vi "1_SimpleDemo_TH260Histo.vi"() -> ()   [LabVIEW 2017]
uses:
  _lib/PQ/TimeHarp260/TH260_MeasMode.ctl
  _lib/PQ/TimeHarp260/TH260_TimingMode.ctl
  _lib/PQ/TimeHarp260/th260lib_x86_x64_UIThread.llb/TH260_DllPath_global.vi
  <vilib>/Utility/error.llb/Error Cluster From Error Code.vi
  _lib/PQ/TimeHarp260/TH260_LibVersion_global.vi
  <vilib>/ErrorRing/Error Ring.xnode
panel:
  in  "dtcode":i32(ring) caption="Deadtime  [ns]" items=["24", "44", "66", "88", "112", "135", "160", "180"]
  in  "TrgLevel":i32=-100 caption="Trg.Level [mV]" min=-1200 max=1200 step=1
  in  "TrgEdge":i32(ring) items=["falling", "rising"]
  in  "SyncTrgEdge":i32(ring) caption="TrgEdge" items=["falling", "rising"]
  in  "SyncTrgLevel":i32=-100 caption="Trg.Level [mV]" min=-1200 max=1200 step=1
  in  "Binning":i32(ring) caption="Resolution [ps]" items=["25.000000", "50.000000", "100.000000", "200.000000", "400.000000", "800.000000", "1600.000000", "3200.000000", "6400.000000", "12800.000000", "25600.000000", "51200.000000", "102400.000000", "204800.000000", "409600.000000", "819200.000000", "1638400.000000", "3276800.000000", "6553600.000000", "13107200.000000", "26214400.000000", "52428800.000000"]
  in  "HistoLength":i32(ring)=5 caption="Histo Length" items=["1024", "2048", "4096", "8192", "16384", "32768"]
  in  "Acqu.Time":i32=10000 caption="Acqu.Time [ms]" min=1 max=360000000 step=1
  in  "GlobalOffset":i32 caption="GlobalOffset [ns]" min=0 max=100000000 step=1
  in  "OverflowLevel":u32=65535 min=1 step=1
  in  "StopOnOverflow":bool=TRUE
  in  "InputZeroX":i32=-10 caption="ZeroCr. [mV]" min=-40 max=0 step=1
  in  "InputCFDLevel":i32=-100 caption="CFDLevel [mV]" min=-1200 max=0 step=1
  in  "Offset":i32 caption="Offset [ps]" min=-99999 max=99999 step=1
  in  "Enable":bool=TRUE
  in  "SyncZeroX":i32=-10 caption="ZeroCr. [mV]" min=-40 max=0 step=1
  in  "SyncCFDLevel":i32=-100 caption="CFDLevel [mV]" min=-1200 max=0 step=1
  in  "SyncOffset":i32 caption="SyncOffset [ps]" min=-99999 max=99999 step=1
  in  "SyncDivider":i32(ring)=8 items=["1"=1, "2"=2, "4"=4, "8"=8]
  out "HistoGraph":T1(graph)={0.0, "Resolution"=0.025, "Histogram"=array2x32768[65536 elements]}
  out "CountRates":i32[](array[numeric]) caption="Count Rates [cps]"
  out "SyncRate":i32 caption="Sync Rate [cps]"
  in  "stop":bool
  out "error out":errorcluster
  # "Acquisition"
  # "All Channels"
  # "Sync"
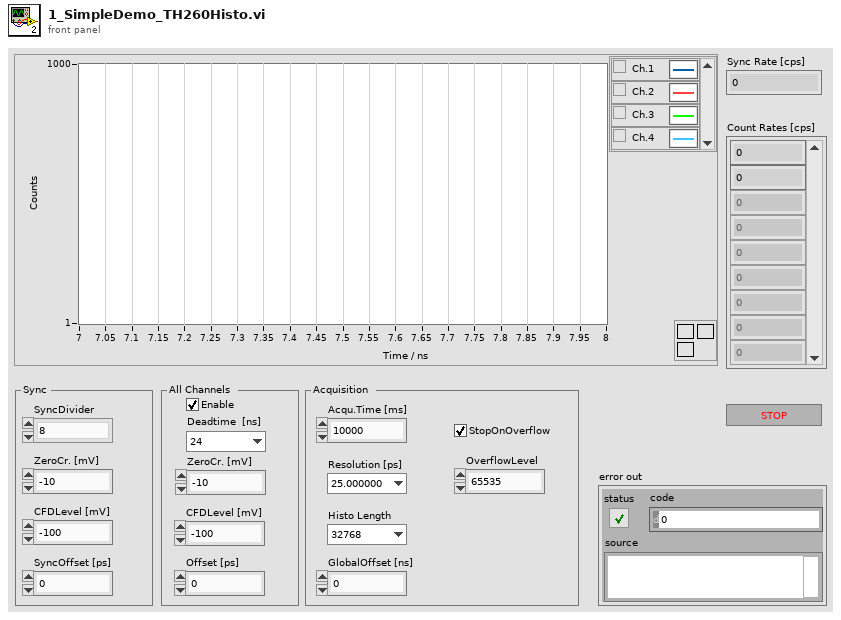
[diagram p1: front panel]
types:
  T1 = cluster{dbl, "Resolution":dbl, "Histogram":u32[][]}
  T2 = typedef "TH260_TimingMode.ctl" = i32
  T3 = typedef "TH260_MeasMode.ctl" = i32
  T4 = typedef "TH260_InitInfo.ctl" = cluster{"Library Version":string, "Serial No.":string, "Model":string, "Partnum":string, "Version":string, "features":i32, "nchannels":i32, "Base Resolution":dbl, "Bin Steps":i32}
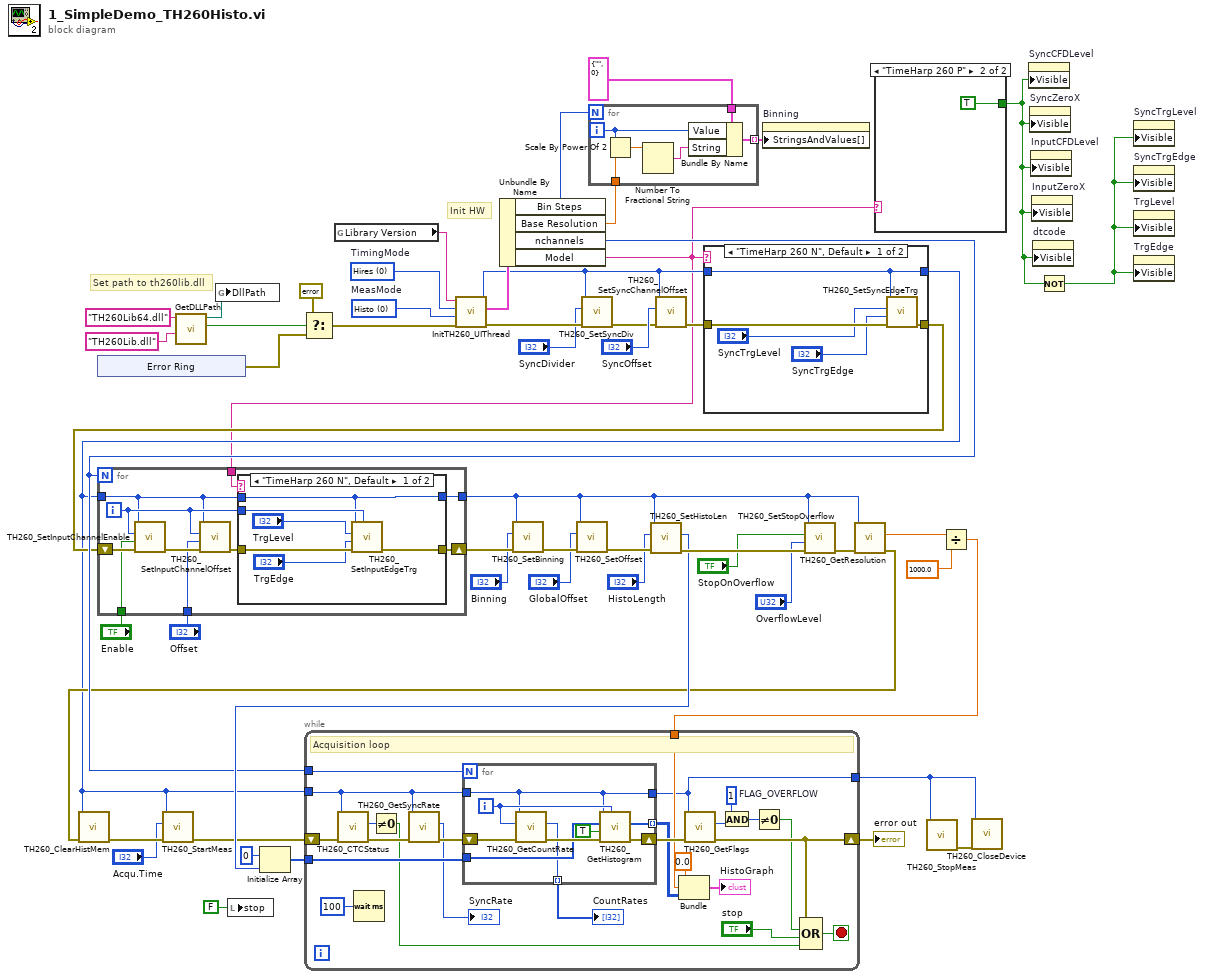
[diagram p0: block diagram]
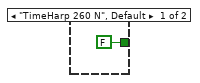
[diagram p2: hidden frame]
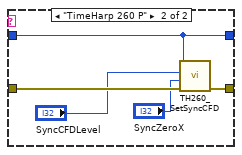
[diagram p3: hidden frame]
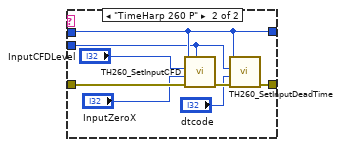
[diagram p4: hidden frame]
diagram:
  w4 = T2 0 items=["Hires", "Lowres"]  # TimingMode
  w54 = T3 0 items=["Histo"=0, "T2"=2, "T3"=3]  # MeasMode
  # "Init HW"
  # "Set path to th260lib.dll"
  n1 = xnode "Error Ring"() -> ("error out"=w53:errorcluster)
  n2 = call "GetDLLPath.vi"("DllName_32bit"="TH260Lib.dll" ("name or relative path"), "DllName_64bit"="TH260Lib64.dll" ("name or relative path")) -> ("file exists?"=w51:bool, "DLLPath"=w50:path)  [unwired: 8 in]
  n3 = global write "TH260_DllPath_global.vi" "DllPath"(w50) -> ()
  n4 = local write "stop"(FALSE ("stop")) -> ()
  n5 = Select(t=errorcluster {"status"=FALSE, "code"=0, "source"=""} ("error IO"), s=w51, f=w53) -> (s? t:f=w47:errorcluster)
  n6 = global read "TH260_LibVersion_global.vi" "Library Version"() -> (w12:string)
  n7 = call "InitTH260_UIThread.vi"("error in (no error)"=w47, "MeasMode"=w54, "TimingMode"=w4, "Library Version"=w12) -> ("error out"=w42:errorcluster, "Init Info"=w44:T4, "DevIdx"=w16:i32)  [unwired: 5 in]
  n8 = Unbundle By Name(w44) -> ("Bin Steps"=w8:i32, "Base Resolution"=w5:dbl, "nchannels"=w24:i32, "Model"=w3:string)
  n9 = call "TH260_SetSyncDiv.vi"("error in (no error)"=w42, "SyncDivider"="SyncDivider", "devidx"=w16) -> ("error out"=w41:errorcluster)  [unwired: 7 in, 1 out]
  n10 = for {
    N: w8 -> [_]
    tunnel: cluster{"String":string, "Value":i32} {"String"="", "Value"=0} -> [w60]
    tunnel: [w59] -> w6 mode=indexing
    tunnel: w5 -> [w58]
    i -> [w57]
    n11 = Scale By Power Of 2(n=w57, x=w58) -> (x*2^n=w56:dbl)
    n12 = Number To Fractional String(number=w56) -> (F-format string=w55:string)  [unwired: 3 in]
    n13 = Bundle By Name(cluster=w60, "Value"=w57, "String"=w55) -> (w59:cluster{"String":string, "Value":i32})
  }
  n14 = call "TH260_SetSyncChannelOffset.vi"("error in (no error)"=w41, "Offset"="SyncOffset", "devidx"=w16) -> ("error out"=w45:errorcluster)  [unwired: 7 in, 1 out]
  n15 = case shown="\"TimeHarp 260 N\", Default" w3 {
    tunnel: w45 -> [w65 w70]
    tunnel: [w64 w68] -> w23
    tunnel: w16 -> [w63 w66]
    tunnel: [w63 w66] -> w9
    frame "TimeHarp 260 N", Default {
      n16 = call "TH260_SetSyncEdgeTrg.vi"("error in (no error)"=w65, "edge"="SyncTrgEdge", "level"="SyncTrgLevel", "devidx"=w63) -> ("error out"=w64:errorcluster)  [unwired: 6 in, 1 out]
    }
    frame "TimeHarp 260 P" {
      n17 = call "TH260_SetSyncCFD.vi"("error in (no error)"=w70, "CFD ZeroCross"="SyncZeroX", "CFD Level"="SyncCFDLevel", "devidx"=w66) -> ("error out"=w68:errorcluster)  [unwired: 6 in, 1 out]
    }
  }
  n18 = for {
    N: w24 -> [_]
    shift-right: [w77] -> w43
    shift-left: w23 -> [w80]
    tunnel: w9 -> [w75]
    tunnel: [w72] -> w19
    tunnel: "Enable" -> [w74]
    tunnel: "Offset" -> [w73]
    tunnel: w3 -> [w71]
    i -> [w76]
    n19 = call "TH260_SetInputChannelEnable.vi"("error in (no error)"=w80, "enable"=w74, "channel"=w76, "devidx"=w75) -> ("error out"=w79:errorcluster)  [unwired: 6 in, 1 out]
    n20 = call "TH260_SetInputChannelOffset.vi"("error in (no error)"=w79, "offset"=w73, "channel"=w76, "devidx"=w75) -> ("error out"=w78:errorcluster)  [unwired: 6 in, 1 out]
    n21 = case shown="\"TimeHarp 260 N\", Default" w71 {
      tunnel: w78 -> [w86 w94]
      tunnel: [w85 w90] -> w77
      tunnel: w76 -> [w84 w88]
      tunnel: w75 -> [w83 w89]
      tunnel: [w83 w89] -> w72
      frame "TimeHarp 260 N", Default {
        n22 = call "TH260_SetInputEdgeTrg.vi"("channel"=w84, "error in (no error)"=w86, "edge"="TrgEdge", "level"="TrgLevel", "devidx"=w83) -> ("error out"=w85:errorcluster)  [unwired: 5 in, 1 out]
      }
      frame "TimeHarp 260 P" {
        n23 = call "TH260_SetInputCFD.vi"("channel"=w88, "error in (no error)"=w94, "CFD ZeroCross"="InputZeroX", "CFD Level"="InputCFDLevel", "devidx"=w89) -> ("error out"=w91:errorcluster)  [unwired: 5 in, 1 out]
        n24 = call "TH260_SetInputDeadTime.vi"("error in (no error)"=w91, "dtcode"="dtcode", "channel"=w88, "devidx"=w89) -> ("error out"=w90:errorcluster)  [unwired: 6 in, 1 out]
      }
    }
  }
  n25 = call "TH260_SetBinning.vi"("error in (no error)"=w43, "Binning"="Binning", "devidx"=w19) -> ("error out"=w39:errorcluster)  [unwired: 7 in, 1 out]
  n26 = call "TH260_SetOffset.vi"("error in (no error)"=w39, "Offset"="GlobalOffset", "devidx"=w19) -> ("error out"=w37:errorcluster)  [unwired: 7 in, 1 out]
  n27 = call "TH260_SetHistoLen.vi"("error in (no error)"=w37, "lencode"="HistoLength", "devidx"=w19) -> ("error out"=w36:errorcluster, "actuallen"=w29:i32)  [unwired: 6 in, 1 out]
  n28 = Initialize Array(u32 0, w29) -> (w28:u32[])
  n29 = property on="Binning" class="Ring (strict)"("StringsAndValues[]"=w6) -> ()  [unwired: 2 in, 2 out]
  n30 = call "TH260_SetStopOverflow.vi"("error in (no error)"=w36, "stopcount"="OverflowLevel", "StopOnOverflow"="StopOnOverflow", "devidx"=w19) -> ("error out"=w20:errorcluster)  [unwired: 6 in, 1 out]
  n31 = call "TH260_GetResolution.vi"("error in (no error)"=w20, "devidx"=w19) -> ("error out"=w17:errorcluster, "resolution"=w18:dbl)  [unwired: 7 in, 1 out]
  n32 = call "TH260_ClearHistMem.vi"("error in (no error)"=w17, "devidx"=w9) -> ("error out"=w33:errorcluster)  [unwired: 8 in, 1 out]
  n33 = call "TH260_StartMeas.vi"("error in (no error)"=w33, "Acquisition time"="Acqu.Time", "devidx"=w9) -> ("error out"=w15:errorcluster)  [unwired: 7 in, 1 out]
  n34 = case shown="\"TimeHarp 260 P\"" w3 {
    tunnel: [FALSE ("Visible") TRUE ("Visible")] -> w2
    frame "TimeHarp 260 N", Default {
    }
    frame "TimeHarp 260 P" {
    }
  }
  n35 = Divide(x=w18, y=1000.0) -> (x/y=w25:dbl)
  n36 = while {
    shift-right: [w108] -> w31
    shift-left: w15 -> [w119]
    tunnel: w9 -> [w115]
    tunnel: w24 -> [w118]
    tunnel: w28 -> [w110]
    tunnel: w25 -> [w102]
    tunnel: [w97] -> w11
    stop <- w109 stop-if-true
    w113 = 1  # FLAG_OVERFLOW
    # "Acquisition loop"
    n37 = call "TH260_CTCStatus.vi"("error in (no error)"=w119, "devidx"=w115) -> ("error out"=w117:errorcluster, "ctcstatus"=w120:i32)  [unwired: 7 in, 1 out]
    n38 = Wait (ms)(milliseconds to wait=u32 100) -> ()  [unwired: 1 out]
    n39 = Not Equal To 0?(x=w120) -> (x != 0?=w99:bool)
    n40 = call "TH260_GetSyncRate.vi"("error in (no error)"=w117, "devidx"=w115) -> ("error out"=w116:errorcluster, "rate"=→"SyncRate":i32)  [unwired: 7 in, 1 out]
    n41 = for {
      N: w118 -> [_]
      shift-right: [w129] -> w114
      shift-left: w116 -> [w128]
      tunnel: w115 -> [w125]
      tunnel: [w125] -> w97
      tunnel: w110 -> [w124]
      tunnel: [w123] -> w105 mode=indexing
      tunnel: [w122] -> w104 mode=indexing
      i -> [w126]
      n42 = call "TH260_GetCountRate.vi"("error in (no error)"=w128, "Channel"=w126, "devidx"=w125) -> ("error out"=w127:errorcluster, "rate"=w123:i32)  [unwired: 6 in, 1 out]
      n43 = call "TH260_GetHistogram.vi"("devidx"=w125, "Buffer"=w124, "clear"=TRUE, "error in (no error)"=w127, "channel"=w126) -> ("Histogram"=w122:u32[], "error out"=w129:errorcluster)  [unwired: 3 in, 1 out]
    }
    "CountRates" <- w105
    n44 = Bundle(0.0, w102, "Histogram"=w104) -> (→"HistoGraph":cluster{dbl, dbl, "Histogram":u32[][]})  [unwired: 1 in]
    n45 = call "TH260_GetFlags.vi"("error in (no error)"=w114, "devidx"=w97) -> ("error out"=w108:errorcluster, "flags"=w111:i32)  [unwired: 7 in, 1 out]
    n46 = And(x=w113, y=w111) -> (x .and. y?=w112:i32)
    n47 = Not Equal To 0?(x=w112) -> (x != 0?=w107:bool)
    n48 = Compound Arithmetic op=OR(w108, w107, "stop", w99) -> (w109:bool)
  }
  "error out" <- w31
  n49 = call "TH260_StopMeas.vi"("devidx"=w11) -> ("error out"=w10:errorcluster)  [unwired: 9 in, 1 out]
  n50 = call "TH260_CloseDevice.vi"("error in (no error)"=w10, "devidx"=w11) -> ()  [unwired: 8 in, 2 out]
  n51 = property on="SyncCFDLevel" class="DigNum (strict)"("Visible"=w2) -> ()  [unwired: 2 in, 2 out]
  n52 = property on="SyncZeroX" class="DigNum (strict)"("Visible"=w2) -> ()  [unwired: 2 in, 2 out]
  n53 = property on="InputCFDLevel" class="DigNum (strict)"("Visible"=w2) -> ()  [unwired: 2 in, 2 out]
  n54 = property on="InputZeroX" class="DigNum (strict)"("Visible"=w2) -> ()  [unwired: 2 in, 2 out]
  n55 = property on="dtcode" class="Ring (strict)"("Visible"=w2) -> ()  [unwired: 2 in, 2 out]
  n56 = Not(x=w2) -> (.not. x?=w1:bool)
  n57 = property on="SyncTrgLevel" class="DigNum (strict)"("Visible"=w1) -> ()  [unwired: 2 in, 2 out]
  n58 = property on="SyncTrgEdge" class="Ring (strict)"("Visible"=w1) -> ()  [unwired: 2 in, 2 out]
  n59 = property on="TrgLevel" class="DigNum (strict)"("Visible"=w1) -> ()  [unwired: 2 in, 2 out]
  n60 = property on="TrgEdge" class="Ring (strict)"("Visible"=w1) -> ()  [unwired: 2 in, 2 out]
